vi "DHE_power.vi"(0 "fd":i32, 7 "flag":i16, 11 "error in (no error)":errorcluster) -> (4 "fd out":i32, 8 "return value":i32, 15 "error out":errorcluster)   [LabVIEW 2016]
doc: "This VI turns instrument power on (Flag=1) or off (Flag=0)."
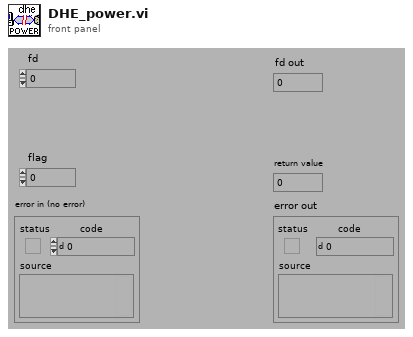
[diagram p1: front panel]
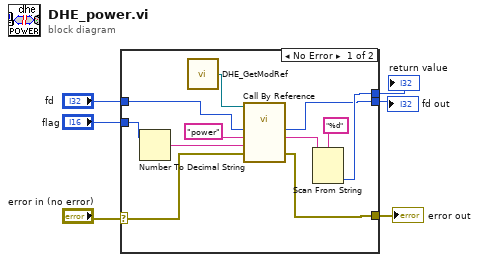
[diagram p0: block diagram]
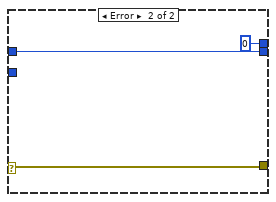
[diagram p2: hidden frame]
diagram:
  n1 = case shown="No Error" "error in (no error)" {
    selector: "error in (no error)" -> [w12 w18]
    tunnel: "fd" -> [w13 w20]
    tunnel: [w10 0] -> w5
    tunnel: [w11 w18] -> w4
    tunnel: "flag" -> [w8 _]
    tunnel: [w9 w20] -> w2
    frame No Error {
      n2 = Number To Decimal String(number=w8) -> (decimal integer string=w7:string)  [unwired: 1 out]
      n3 = call "DHE_GetModRef.vi"() -> ("DHE_ModRef"=w17:refnum<vi>)  [unwired: 9 out]
      n4 = call-by-ref "?"(reference=w17, "error in (no error)"=w12, "arguments"=w7, "function"="power", "fd in"=w13) -> ("error out"=w11:errorcluster, "str result"=w15:string, "fd out"=w9:i32)  [unwired: 5 in, 3 out]
      n5 = Scan From String(format string="%d", input string=w15) -> (output 1=w10:i32)  [unwired: 2 in, 4 out]
    }
    frame Error {
    }
  }
  "error out" <- w4
  "return value" <- w5
  "fd out" <- w2
